vi "ButtonPutToteDown.vi"(11 "POVs":i16[](array[numeric])) -> ()   [LabVIEW 2014]
uses:
  Gantry/GantryGlobals.vi
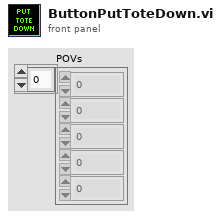
[diagram p1: front panel]
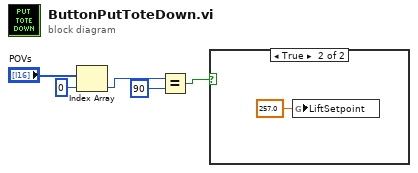
[diagram p0: block diagram]
diagram:
  n1 = Index Array(array="POVs", index=0) -> (element=w3:i16)
  n2 = Equal?(x=w3, y=i16 90) -> (x = y?=w1:bool)
  n3 = case shown="True" w1 {
    frame False {
    }
    frame True {
      n4 = global write "GantryGlobals.vi" "LiftSetpoint"(257.0 ("LiftSetpoint")) -> ()
    }
  }
